vi "Config Folder.vi"(8 "error in (no error)":errorcluster, 11 "Git Updater Module in":refnum<class "Git Updater Module.lvclass">) -> (0 "error out":errorcluster, 2 "Config Folder":path, 3 "Git Updater Module out":refnum<class "Git Updater Module.lvclass">)   [LabVIEW 2020, in "VolatusGUI.lvlib" / "Git Updater Module.lvclass"]
uses:
  Git Updater Module.lvclass
  Git Updater Module.lvclass/Git Updater Module.ctl
  Volatus/Module/Module.lvclass
  Volatus/VolatusAPI/VolatusAPI.lvclass
  C:/dev/lv20CE/relink/lv-volatus/Volatus/Module/Module.lvclass
  C:/dev/lv20CE/relink/lv-volatus/VolatusGUI/Git Updater Module/Git Updater Module.lvclass
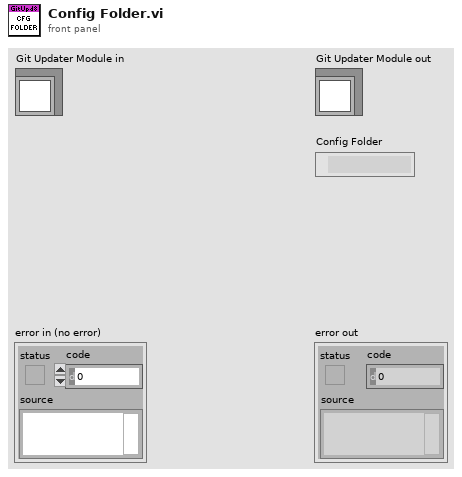
[diagram p1: front panel]
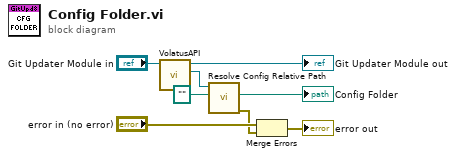
[diagram p0: block diagram]
diagram:
  n1 = call "VolatusAPI.vi"("Module in"="Git Updater Module in") -> ("VolatusAPI"=w7:refnum<class "VolatusAPI.lvclass">, "Module out"=→"Git Updater Module out":refnum<class "Git Updater Module.lvclass">)  [unwired: 9 in]
  n2 = call "Resolve Config Relative Path.vi"("Path"=path "", "VolatusAPI in"=w7) -> ("error out"=w1:errorcluster, "Resolved Path"=→"Config Folder":path)  [unwired: 7 in, 1 out]
  n3 = Merge Errors("error in (no error)", w1) -> (→"error out":errorcluster)
